vi "Read Value.vi"(8 "error in (no error)":errorcluster, 10 "Key":i32, 11 "Integer Dictionary in":refnum<class "Integer Dictionary.lvclass">) -> (0 "error out":errorcluster, 1 "Value":variant, 2 "found?":bool, 3 "Integer Dictionary out":refnum<class "Integer Dictionary.lvclass">)   [LabVIEW 2013, in "Integer Dictionary.lvclass"]
uses:
  Integer Dictionary.lvclass
  Integer Dictionary.lvclass/Integer Dictionary.ctl
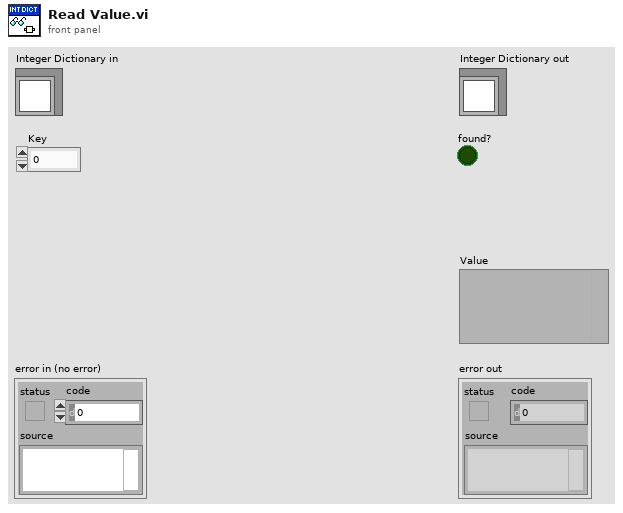
[diagram p1: front panel]
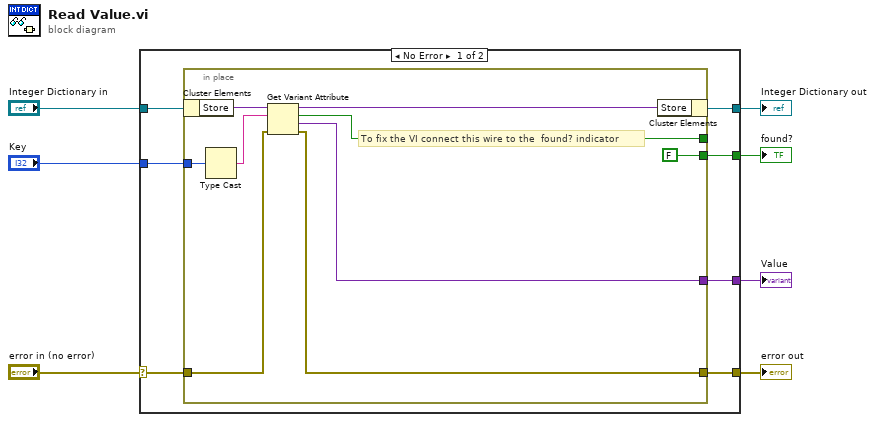
[diagram p0: block diagram]
diagram:
  n1 = case shown="No Error" "error in (no error)" {
    selector: "error in (no error)" -> [w12 w25]
    tunnel: [w11 w25] -> w6
    tunnel: [w13 w24] -> w4
    tunnel: "Integer Dictionary in" -> [w14 w24]
    tunnel: "Key" -> [w10 _]
    tunnel: [w9 _] -> w2
    tunnel: [w8 _] -> w1
    frame No Error {
      n2 = in-place {
        in-place-border: w12 -> [w21]
        in-place-border: [w20] -> w11
        in-place-border: w10 -> [w19]
        in-place-border: [FALSE] -> w9
        in-place-border: [w17] -> w8
        in-place-border: [w15] -> _
        # "To fix the VI connect this wire to the  found? indicator"
        n3 = in-place-cluster #1(w14) -> ("Store"=w23:variant)
        n4 = Type Cast(x=w19) -> (*(type *) &x=w18:string)  [unwired: 1 in]
        n5 = Get Variant Attribute(Variant=w23, name=w18, error in=w21) -> (duplicate Variant=w22:variant, found=w15:bool, value=w17:variant, error out=w20:errorcluster)  [unwired: 1 in]
        n6 = in-place-cluster #1("Store"=w22) -> (w13:refnum<class "Integer Dictionary.lvclass">)
      }
    }
    frame Error {
    }
  }
  "error out" <- w6
  "Integer Dictionary out" <- w4
  "found?" <- w2
  "Value" <- w1
